vi "Update Value.vi"(6 "Time":dbl, 8 "error in (no error)":errorcluster, 11 "BooleanControl in":refnum<class "BooleanControl.lvclass">) -> (0 "error out":errorcluster, 1 "Update":bool, 2 "Value":variant, 3 "BooleanControl out":refnum<class "BooleanControl.lvclass">)   [LabVIEW 2020, in "VolatusGUIElements.lvlib" / "BooleanControl.lvclass"]
uses:
  BooleanControl.lvclass
  BooleanControl.lvclass/BooleanControl.ctl
  lv-vecto/Vecto/Channel DBL/Channel DBL.lvclass/Channel DBL.ctl
  lv-vecto/Vecto/Group DBL/Value by Index.vi
  lv-vecto/Vecto/Channel DBL/Channel DBL.lvclass
  VolatusGUIElements.lvlib
  lv-vecto/Vecto/Vecto.lvlib
  VolatusGUI/Element Inhibit/Element Inhibit.lvclass
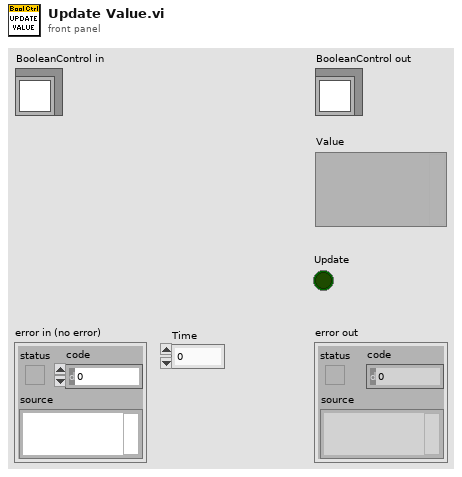
[diagram p1: front panel]
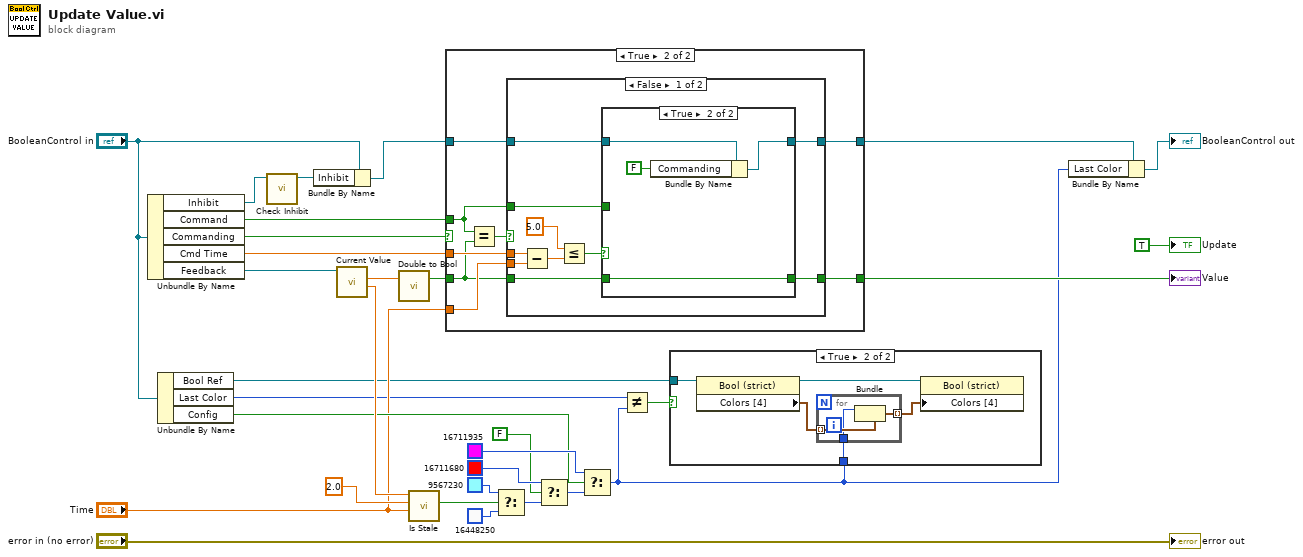
[diagram p0: block diagram]
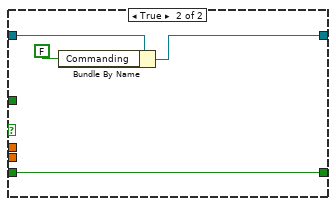
[diagram p4: hidden frame]
diagram:
  n1 = Unbundle By Name("BooleanControl in") -> ("Inhibit"=w3:refnum<class "Element Inhibit.lvclass">, "Command"=w16:bool, "Commanding"=w28:bool, "Cmd Time"=w26:dbl, "Feedback"=w30:refnum<class "Channel DBL.lvclass">)
  n2 = Unbundle By Name("BooleanControl in") -> ("Bool Ref"=w6:refnum<vi>, "Last Color"=w8:u32, "Config"=w17:bool)
  n3 = call "Check Inhibit.vi"("Element Inhibit in"=w3) -> ("Element Inhibit out"=w1:refnum<class "Element Inhibit.lvclass">)  [unwired: 9 in, 1 out]
  n4 = Bundle By Name(cluster="BooleanControl in", "Inhibit"=w1) -> (w2:refnum<class "BooleanControl.lvclass">)
  n5 = call "Current Value.vi"("Channel in"=w30) -> ("Timestamp"=w29:dbl, "Scaled"=w27:dbl)  [unwired: 6 in, 3 out]
  n6 = call "Double to Bool.vi"("Double"=w27) -> ("Bool"=w25:bool)  [unwired: 2 in]
  n7 = call "Is Stale.vi"("Time"="Time", "Staleness"=2.0, "Timestamp"=w29) -> ("Stale"=w24:bool)  [unwired: 8 in]
  n8 = case shown="True" w28 {
    tunnel: w25 -> [w33 w38]
    tunnel: w26 -> [_ w41]
    tunnel: "Time" -> [_ w40]
    tunnel: w16 -> [_ w34]
    tunnel: w2 -> [w32 w37]
    tunnel: [w32 w36] -> w12
    tunnel: [w33 w35] -> w10
    frame False {
    }
    frame True {
      n9 = Equal?(x=w34, y=w38) -> (x = y?=w39:bool)
      n10 = case shown="False" w39 {
        tunnel: w41 -> [w51 _]
        tunnel: w40 -> [w50 _]
        tunnel: w38 -> [w44 w58]
        tunnel: w37 -> [w46 w61]
        tunnel: [w45 w59] -> w36
        tunnel: [w42 w58] -> w35
        tunnel: w34 -> [w43 _]
        frame False {
          n11 = Subtract(x=w51, y=w50) -> (x-y=w49:dbl)
          n12 = Less Or Equal?(x=5.0, y=w49) -> (x <= y?=w47:bool)
          n13 = case shown="True" w47 {
            tunnel: w46 -> [w52 w57]
            tunnel: [w52 w55] -> w45
            tunnel: w44 -> [_ w54]
            tunnel: w43 -> [w53 _]
            tunnel: [w53 w54] -> w42
            frame False {
            }
            frame True {
              n14 = Bundle By Name(cluster=w57, "Commanding"=FALSE) -> (w55:refnum<class "BooleanControl.lvclass">)
            }
          }
        }
        frame True {
          n15 = Bundle By Name(cluster=w61, "Commanding"=FALSE) -> (w59:refnum<class "BooleanControl.lvclass">)
        }
      }
    }
  }
  "Value" <- w10
  n16 = Select(t=u32 9567230, s=w24, f=u32 16448250) -> (s? t:f=w21:u32)
  n17 = Select(t=u32 16711680, s=FALSE, f=w21) -> (s? t:f=w19:u32)
  n18 = Select(t=u32 16711935, s=w17, f=w19) -> (s? t:f=w4:u32)
  n19 = Not Equal?(x=w8, y=w4) -> (x != y?=w7:bool)
  n20 = case shown="True" w7 {
    tunnel: w6 -> [_ w65]
    tunnel: w4 -> [_ w64]
    frame False {
    }
    frame True {
      n21 = property class="Bool (strict)"(reference=w65) -> (reference out=w63:refnum<vi>, "Colors [4]"=w62:cluster{u32, u32}[])  [unwired: 1 in, 1 out]
      n22 = for {
        tunnel: w62 -> [w69] mode=indexing
        tunnel: [w68] -> w66 mode=indexing
        tunnel: w64 -> [w67]
        n23 = Bundle(cluster=w69, w67) -> (w68:cluster{u32, u32})  [unwired: 1 in]
      }
      n24 = property class="Bool (strict)"(reference=w63, "Colors [4]"=w66) -> ()  [unwired: 1 in, 2 out]
    }
  }
  n25 = Bundle By Name(cluster=w12, "Last Color"=w4) -> (→"BooleanControl out":refnum<class "BooleanControl.lvclass">)
  "error out" <- "error in (no error)"
  "Update" <- TRUE ("Update")
